vi "GetPriceFromWebsite.vi"(3 "Search String":string, 5 "Website In":string) -> (0 "error out":errorcluster, 1 "Result Price":string, 2 "RawData":string)   [LabVIEW 2020]
uses:
  <vilib>/regexp/Match Regular Expression.xnode
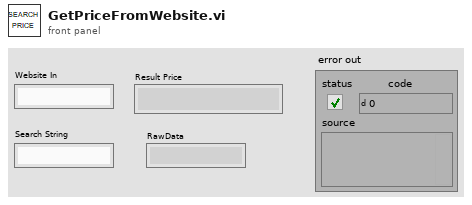
[diagram p1: front panel]
types:
  T1 = enum16{"Read", "Write", "ReadWrite", "BufferedRead", "BufferedReadWrite"}
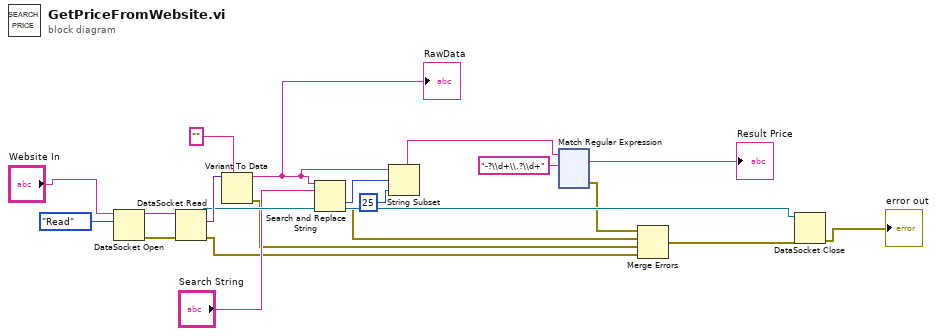
[diagram p0: block diagram]
diagram:
  n1 = DataSocket Open(10:T1."Read" ("mode"), 11:"Website In") -> (0:w12:errorcluster, 3:w13:refnum<k13>)  [unwired: 2 in]
  n2 = DataSocket Read(8:w12, 11:w13) -> (0:w4:errorcluster, 2:w20:variant, 3:w10:refnum<k13>)  [unwired: 3 in, 4 out]
  n3 = Variant To Data(type="", Variant=w20) -> (data=w7:string, error out=w5:errorcluster)  [unwired: 1 in]
  "RawData" <- w7
  n4 = Search and Replace String(input string=w7, search string="Search String") -> (offset past replacement=w18:i32, error out=w3:errorcluster)  [unwired: 6 in, 2 out]
  n5 = String Subset(string=w7, offset (0)=w18, length (rest)=25 ("length (rest)")) -> (substring=w16:string)
  n6 = xnode "Match Regular Expression"("input string"=w16, "regular expression"="-?\\d+\\.?\\d+") -> ("whole match"=→"Result Price":string, "error out"=w2:errorcluster)  [unwired: 4 in, 3 out]
  n7 = Merge Errors(w2, w3, w5, w4) -> (w1:errorcluster)
  n8 = DataSocket Close(8:w1, 11:w10) -> (0:→"error out":errorcluster)  [unwired: 1 in, 1 out]
